vi "ErrDecoder.vi"(1 "err code":dbl) -> (0 "err string":string)   [LabVIEW 2012]
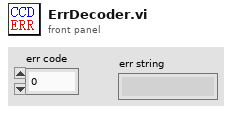
[diagram p1: front panel]
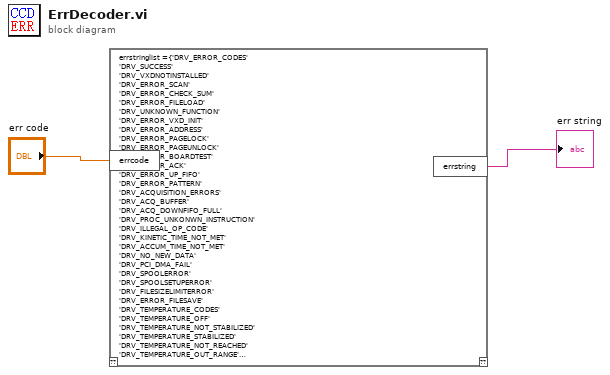
[diagram p0: block diagram]
diagram:
  n1 = script code="errstringlist ={'DRV_ERROR_CODES'\n'DRV_SUCCESS'\n'DRV_VXDNOTINSTALLED'\n'DRV_ERROR_SCAN'\n'DRV_ERROR_CHECK_SUM'\n'DRV_ERROR_FILELOAD'\n'DRV_UNKNOWN_FUNCTION'\n'DRV_ERROR_VXD_INIT'\n'DRV_ERROR_ADDRESS'\n'DRV_ERROR_PAGELOCK'\n'DRV_ERROR_PAGEUNLOCK'\n'DRV_ERROR_BOARDTEST'\n'DRV_ERROR_ACK'\n'DRV_ERROR_UP_FIFO'\n'DRV_ERROR_PATTERN'\n'DRV_ACQUISITION_ERRORS'\n'DRV_ACQ_BUFFER'\n'DRV_ACQ_DOWNFIFO_FULL'\n'DRV_PROC_UNKONWN_INSTRUCTION'\n'DRV_ILLEGAL_OP_CODE'\n'DRV_KINETIC_TIME_NOT_MET'\n'DRV_ACCUM_TIME_NOT_MET'\n'DRV_NO_NEW_DATA'\n'DRV_PCI_DMA_FAIL'\n'DRV_SPOOLERROR'\n'DRV_SPOOLSETUPERROR'\n'DRV_FILESIZELIMITERROR'\n'DRV_ERROR_FILESAVE'\n'DRV_TEMPERATURE_CODES'\n'DRV_TEMPERATURE_OFF'\n'DRV_TEMPERATURE_NOT_STABILIZED'\n'DRV_TEMPERATURE_STABILIZED'\n'DRV_TEMPERATURE_NOT_REACHED'\n'DRV_TEMPERATURE_OUT_RANGE'\n'DRV_TEMPERATURE_NOT_SUPPORTED'\n'DRV_TEMPERATURE_DRIFT'\n'DRV_TEMP_CODES'\n'DRV_TEMP_OFF'\n'DRV_TEMP_NOT_STABILIZED'\n'DRV_TEMP_STABILIZED'\n'DRV_TEMP_NOT_REACHED'\n'DRV_TEMP_OUT_RANGE'\n'DRV_TEMP_NOT_SUPPORTED'\n'DRV_TEMP_DRIFT'\n'DRV_GENERAL_ERRORS'\n'DRV_INVALID_AUX'\n'DRV_COF_NOTLOADED'\n'DRV_FPGAPROG'\n'DRV_FLEXERROR'\n'DRV_GPIBERROR'\n'DRV_EEPROMVERSIONERROR'\n'DRV_DATATYPE'\n'DRV_DRIVER_ERRORS'\n'DRV_P1INVALID'\n'DRV_P2INVALID'\n'DRV_P3INVALID'\n'DRV_P4INVALID'\n'DRV_INIERROR'\n'DRV_COFERROR'\n'DRV_ACQUIRING'\n'DRV_IDLE'\n'DRV_TEMPCYCLE'\n'DRV_NOT_INITIALIZED'\n'DRV_P5INVALID'\n'DRV_P6INVALID'\n'DRV_INVALID_MODE'\n'DRV_INVALID_FILTER'\n'DRV_I2CERRORS'\n'DRV_I2CDEVNOTFOUND'\n'DRV_I2CTIMEOUT'\n'DRV_P7INVALID'\n'DRV_P8INVALID'\n'DRV_P9INVALID'\n'DRV_P10INVALID'\n'DRV_P11INVALID'\n'DRV_USBERROR'\n'DRV_IOCERROR'\n'DRV_VRMVERSIONERROR'\n'DRV_GATESTEPERROR'\n'DRV_USB_INTERRUPT_ENDPOINT_ERROR'\n'DRV_RANDOM_TRACK_ERROR'\n'DRV_INVALID_TRIGGER_MODE'\n'DRV_LOAD_FIRMWARE_ERROR'\n'DRV_DIVIDE_BY_ZERO_ERROR'\n'DRV_INVALID_RINGEXPOSURES'\n'DRV_BINNING_ERROR'\n'DRV_INVALID_AMPLIFIER'\n'DRV_INVALID_COUNTCONVERT_MODE'\n'DRV_ERROR_NOCAMERA'\n'DRV_NOT_SUPPORTED'\n'DRV_NOT_AVAILABLE'\n'DRV_ERROR_MAP'\n'DRV_ERROR_UNMAP'\n'DRV_ERROR_MDL'\n'DRV_ERROR_UNMDL'\n'DRV_ERROR_BUFFSIZE'\n'DRV_ERROR_NOHANDLE'\n'DRV_GATING_NOT_AVAILABLE'\n'DRV_FPGA_VOLTAGE_ERROR'\n'DRV_OW_CMD_FAIL'\n'DRV_OWMEMORY_BAD_ADDR'\n'DRV_OWCMD_NOT_AVAILABLE'\n'DRV_OW_NO_SLAVES'\n'DRV_OW_NOT_INITIALIZED'\n'DRV_OW_ERROR_SLAVE_NUM'\n'DRV_MSTIMINGS_ERROR'\n'DRV_OA_NULL_ERROR'\n'DRV_OA_PARSE_DTD_ERROR'\n'DRV_OA_DTD_VALIDATE_ERROR'\n'DRV_OA_FILE_ACCESS_ERROR'\n'DRV_OA_FILE_DOES_NOT_EXIST'\n'DRV_OA_XML_INVALID_OR_NOT_FOUND_ERROR'\n'DRV_OA_PRESET_FILE_NOT_LOADED'\n'DRV_OA_USER_FILE_NOT_LOADED'\n'DRV_OA_PRESET_AND_USER_FILE_NOT_LOADED'\n'DRV_OA_INVALID_FILE'\n'DRV_OA_FILE_HAS_BEEN_MODIFIED'\n'DRV_OA_BUFFER_FULL'\n'DRV_OA_INVALID_STRING_LENGTH'\n'DRV_OA_INVALID_CHARS_IN_NAME'\n'DRV_OA_INVALID_NAMING'\n'DRV_OA_GET_CAMERA_ERROR'\n'DRV_OA_MODE_ALREADY_EXISTS'\n'DRV_OA_STRINGS_NOT_EQUAL'\n'DRV_OA_NO_USER_DATA'\n'DRV_OA_VALUE_NOT_SUPPORTED'\n'DRV_OA_MODE_DOES_NOT_EXIST'\n'DRV_OA_CAMERA_NOT_SUPPORTED'\n'DRV_OA_FAILED_TO_GET_MODE'\n'DRV_PROCESSING_FAILED'\n};\n\nerrlist = [20001\n20002\n20003\n20004\n20005\n20006\n20007\n20008\n20009\n20010\n20011\n20012\n20013\n20014\n20015\n20017\n20018\n20019\n20020\n20021\n20022\n20023\n20024\n20025\n20026\n20027\n20028\n20029\n20033\n20034\n20035\n20036\n20037\n20038\n20039\n20040\n20033\n20034\n20035\n20036\n20037\n20038\n20039\n20040\n20049\n20050\n20051\n20052\n20053\n20054\n20055\n20064\n20065\n20066\n20067\n20068\n20069\n20070\n20071\n20072\n20073\n20074\n20075\n20076\n20077\n20078\n20079\n20080\n20081\n20082\n20083\n20084\n20085\n20086\n20087\n20089\n20090\n20091\n20092\n20093\n20094\n20095\n20096\n20097\n20098\n20099\n20100\n20101\n20990\n20991\n20992\n20115\n20116\n20117\n20118\n20119\n20121\n20130\n20131\n20150\n20151\n20152\n20153\n20154\n20155\n20156\n20173\n20174\n20175\n20176\n20177\n20178\n20179\n20180\n20181\n20182\n20183\n20184\n20185\n20186\n20187\n20188\n20189\n20190\n20191\n20192\n20193\n20194\n20195\n20211\n];\n\nindex = find(errlist == errcode);\nif(~isempty(index))\n\terrstring = errstringlist{index(1)};\nelse\n\terrstring = 'unknown error';\nend"("errcode"="err code") -> ("errstring"=→"err string":string)  [unwired: 1 in, 1 out]
